vi "CalculateImageSize.vi"(8 "error in (no error)":errorcluster, 10 "String":string, 11 "EAN-13 in":refnum<class "EAN-13.lvclass">) -> (0 "error out":errorcluster, 2 "Size":cluster{"x":i16, "y":i16}, 3 "EAN-13 out":refnum<class "EAN-13.lvclass">)   [LabVIEW 2013, in "BarCodes.lvlib" / "EAN-13.lvclass"]
doc: "Calculates the size of the image for the barcode. This should include the entire barcode, quiet space, and text around it."
uses:
  EAN-13.lvclass
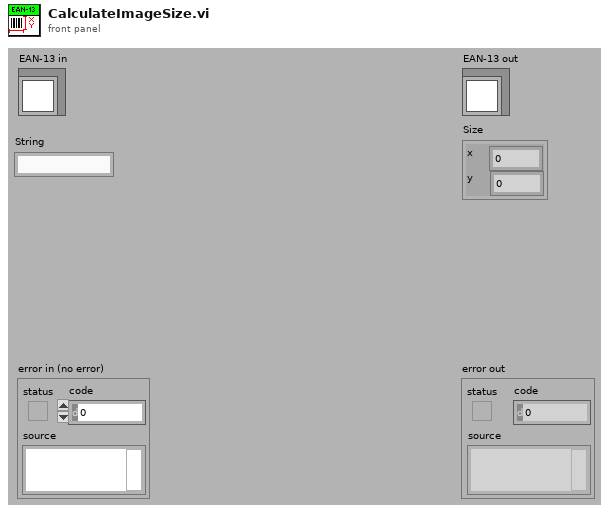
[diagram p1: front panel]
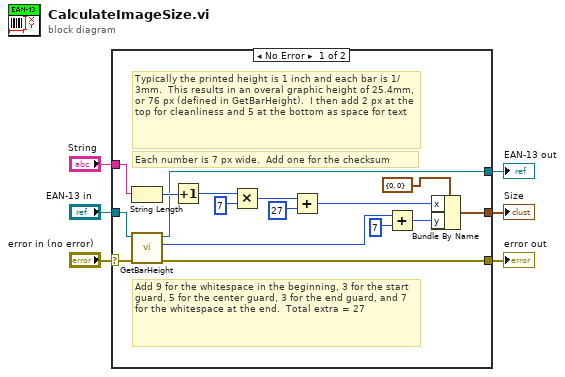
[diagram p0: block diagram]
diagram:
  n1 = case shown="No Error" "error in (no error)" {
    selector: "error in (no error)" -> [w7 w23]
    tunnel: "String" -> [w22 _]
    tunnel: "EAN-13 in" -> [w14 w24]
    tunnel: [w13 w24] -> w4
    tunnel: [w12 w23] -> w3
    tunnel: [w8 _] -> w2
    frame No Error {
      # "Typically the printed height is 1 inch and each bar is 1/3mm.  This results in an overal graphic height of 25.4mm, or 76 px (defined in GetBarHeight).  I then add 2 px at the top for cleanliness and 5 at the bottom as space for text"
      # "Add 9 for the whitespace in the beginning, 3 for the start guard, 5 for the center guard, 3 for the end guard, and 7 for the whitespace at the end.  Total extra = 27"
      # "Each number is 7 px wide.  Add one for the checksum"
      n2 = String Length(string=w22) -> (length=w21:i32)
      n3 = call-dynamic "GetBarHeight.vi"("error in (no error)"=w7, "EAN-13 in"=w14) -> ("error out"=w12:errorcluster, "Bar Height"=w11:u8, "EAN-13 out"=w13:refnum<class "EAN-13.lvclass">)  [unwired: 7 in]
      n4 = Increment(x=w21) -> (x+1=w17:i32)
      n5 = Multiply(x=w17, y=7) -> (x*y=w19:i32)
      n6 = Add(x=w19, y=27) -> (x+y=w15:i32)
      n7 = Add(x=w11, y=i16 7) -> (x+y=w9:i16)
      n8 = Bundle By Name(cluster=cluster{"x":i16, "y":i16} {"x"=0, "y"=0} ("Size"), "x"=w15, "y"=w9) -> (w8:cluster{"x":i16, "y":i16})
    }
    frame Error {
    }
  }
  "error out" <- w3
  "EAN-13 out" <- w4
  "Size" <- w2
